vi "Elapsed Time.vi"(10 "Target (ms)":u32=500, 11 "Reset":bool) -> (2 "Elapsed Time Since Reset":u32, 3 "Elapsed":bool)   [LabVIEW 2025, in "I2C Bus Monitor UI.lvlib"]
uses:
  I2C Bus Monitor UI.lvlib
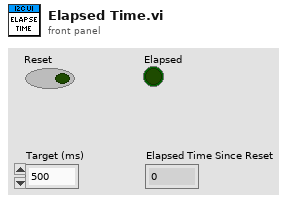
[diagram p1: front panel]
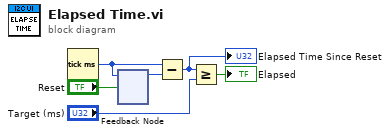
[diagram p0: block diagram]
diagram:
  n1 = Tick Count (ms)() -> (millisecond timer value=w5:u32)
  n2 = feedback #1() -> (w4:u32)  [unwired: 1 in]
  n3 = feedback-in #1(w5, "Reset") -> ()
  n4 = Subtract(x=w5, y=w4) -> (x-y=w3:u32)
  "Elapsed Time Since Reset" <- w3
  n5 = Greater Or Equal?(x=w3, y="Target (ms)") -> (x >= y?=→"Elapsed":bool)
